vi "TankDrive.vi"(8 "Error In (no error)":errorcluster, 9 "Right Motor Value":dbl, 10 "Left Motor Value":dbl, 11 "RobotDriveDevRef":T1={"DevStatus"={"status"=FALSE, "code"=0, "source"=""}, "Motors[]"=[], "Square Inputs"=FALSE, "Max Output"=1.0, "Isochronous"=FALSE}) -> (0 "Error Out":errorcluster)   [LabVIEW 2012]
doc: "Sets the TankDrive motor inputs to the two given values."
uses:
  <vilib>/Rock Robotics/WPI/RobotDrive/WPI_RobotDriveDevRef.ctl
  <vilib>/Rock Robotics/WPI/MotorControl/WPI_MotorControlDeviceRef.ctl
  <vilib>/Rock Robotics/SystemInterfaces/Typedef/FPGA_TypedefDigitalModule.ctl
  <vilib>/Rock Robotics/SystemInterfaces/DIO/FPGA_DIOPWMChannel.ctl
  <vilib>/Rock Robotics/WPI/PWM/WPI_PWMDeadband.ctl
  <vilib>/Rock Robotics/WPI/CAN/Jaguar/SubVIs/WPI_CANJaguar_ControlMode.ctl
  <vilib>/Rock Robotics/WPI/PWM/WPI_PWMTransform_ConPane.ctl
panel:
  in  "HalfSpeed":bool=TRUE
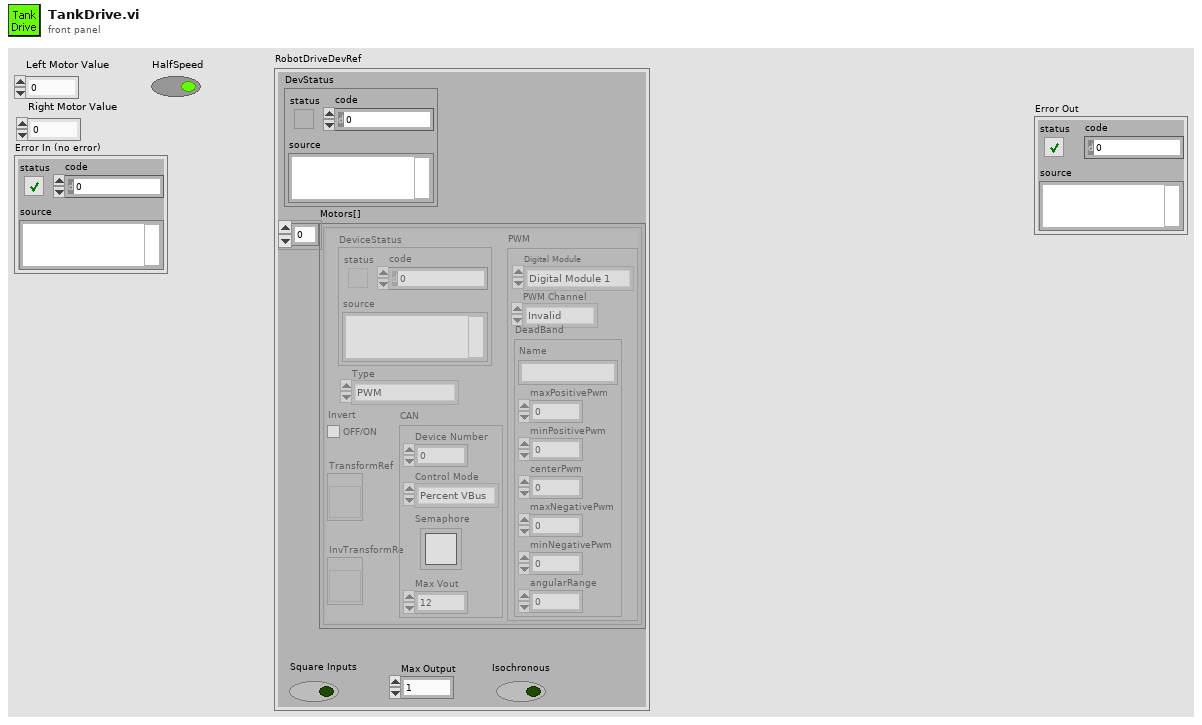
[diagram p1: front panel]
types:
  T1 = typedef "WPI_RobotDriveDevRef.ctl" = cluster{"DevStatus":errorcluster, "Motors[]":T2[], "Square Inputs":bool, "Max Output":dbl, "Isochronous":bool}
  T2 = typedef "WPI_MotorControlDeviceRef.ctl" = cluster{"DeviceStatus":errorcluster, "Type":enum16{"PWM", "CAN"}, "PWM":cluster{"Digital Module":T3, "PWM Channel":T4, "DeadBand":T5}, "CAN":cluster{"Device Number":u8, "Control Mode":T6, "Semaphore":T7, "Max Vout":dbl}, "Invert":bool, "TransformRef":T8, "InvTransformRef":T8}
  T3 = typedef "FPGA_TypedefDigitalModule.ctl" = enum16{"Digital Module 1", "Digital Module 2"}
  T4 = typedef "FPGA_DIOPWMChannel.ctl" = enum8{"PWM 1", "PWM 2", "PWM 3", "PWM 4", "PWM 5", "PWM 6", "PWM 7", "PWM 8", "PWM 9", "PWM 10", "Invalid"}
  T5 = typedef "WPI_PWMDeadband.ctl" = cluster{"Name":string, "maxPositivePwm":i32, "minPositivePwm":i32, "centerPwm":i32, "maxNegativePwm":i32, "minNegativePwm":i32, "angularRange":u16}
  T6 = typedef "WPI_CANJaguar_ControlMode.ctl" = enum8{"Percent VBus", "Current", "Speed", "Position", "Voltage"}
  T7 = typedef "Semaphore RefNum" = refnum<k1>
  T8 = typedef "WPI_PWMTransform_ConPane.ctl" = refnum<vi>
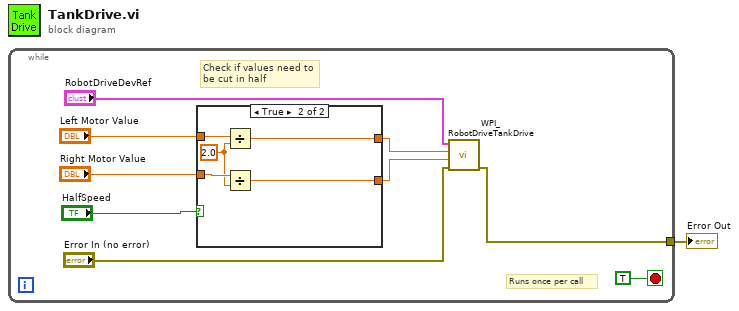
[diagram p0: block diagram]
diagram:
  n1 = while {
    tunnel: [w9] -> w1
    stop <- TRUE stop-if-true
    # "Check if values need to \nbe cut in half"
    # "Runs once per call"
    n2 = case shown="True" "HalfSpeed" {
      tunnel: "Right Motor Value" -> [w12 w16]
      tunnel: "Left Motor Value" -> [w11 w17]
      tunnel: [w11 w14] -> w3
      tunnel: [w12 w13] -> w2
      frame False {
      }
      frame True {
        w15 = 2.0
        n3 = Divide(x=w17, y=w15) -> (x/y=w14:dbl)
        n4 = Divide(x=w16, y=w15) -> (x/y=w13:dbl)
      }
    }
    n5 = call <vilib>:"WPI_RobotDriveTankDrive.vi"("error in (no error)"="Error In (no error)", "Right axis value"=w2, "Left axis value"=w3, "RobotDriveDevRef"="RobotDriveDevRef") -> ("error out"=w9:errorcluster)  [unwired: 5 in, 2 out]
  }
  "Error Out" <- w1
